vi "Excel报表.vi"() -> ()   [LabVIEW 2014]
uses:
  <vilib>/Utility/NIReport.llb/NI_report.lvclass
  <vilib>/Utility/NIReport.llb/Excel/NI_Excel.lvclass
panel:
  in  "template (empty)":path caption="模板（空）"
  in  "Relative Humidity":dbl[][](array[numeric])=[[0.54, 0.65, 0.56, 0.5, 0.45]]
  in  "Has Legend?":bool
  in  "Graph Type":i32(ring)=51 items=["xlColumnClustered"=51, "xlColumnStacked"=52, "xlColumnStacked100"=53, "xl3DColumnClustered"=54, "xl3DColumnStacked"=55, "xl3DColumnStacked100"=56, "xlBarClustered"=57, "xlBarStacked"=58, "xlBarStacked100"=59, "xl3DBarClustered"=60, "xl3DBarStacked"=61, "xl3DBarStacked100"=62, "xlLineStacked"=63, "xlLineStacked100"=64, "xlLineMarkers"=65, "xlLineMarkersStacked"=66, "xlLineMarkersStacked100"=67, "xlPieOfPie"=68, "xlPieExploded"=69, "xl3DPieExploded"=70, "xlBarOfPie"=71, "xlXYScatterSmooth"=72, "xlXYScatterSmoothNoMarkers"=73, "xlXYScatterLines"=74, "xlXYScatterLinesNoMarkers"=75, "xlAreaStacked"=76, "xlAreaStacked100"=77, "xl3DAreaStacked"=78, "xl3DAreaStacked100"=79, "xlDoughnutExploded"=80, "xlRadarMarkers"=81, "xlRadarFilled"=82, "xlSurface"=83, "xlSurfaceWireframe"=84, "xlSurfaceTopView"=85, "xlSurfaceTopViewWireframe"=86, "xlBubble"=15, "xlBubble3DEffect"=87, "xlStockHLC"=88, "xlStockOHLC"=89, "xlStockVHLC"=90, "xlStockVOHLC"=91, "xlCylinderColClustered"=92, "xlCylinderColStacked"=93, "xlCylinderColStacked100"=94, "xlCylinderBarClustered"=95, "xlCylinderBarStacked"=96, "xlCylinderBarStacked100"=97, "xlCylinderCol"=98, "xlConeColClustered"=99, "xlConeColStacked"=100, "xlConeColStacked100"=101, "xlConeBarClustered"=102, "xlConeBarStacked"=103, "xlConeBarStacked100"=104, "xlConeCol"=105, "xlPyramidColClustered"=106, "xlPyramidColStacked"=107, "xlPyramidColStacked100"=108, "xlPyramidBarClustered"=109, "xlPyramidBarStacked"=110, "xlPyramidBarStacked100"=111, "xlPyramidCol"=112, "xl3DColumn"=-4100, "xlLine"=4, "xl3DLine"=-4101, "xl3DPie"=-4102, "xlPie"=5, "xlXYScatter"=-4169, "xl3DArea"=-4098, "xlArea"=1, "xlDoughnut"=-4120, "xlRadar"=-4151]
  in  "Month":string[](array[string])=["Jan", "Feb", "Mar", "Apr", "May"]
  in  "Window State":enum16{"maximized", "minimized", "normal"}(ring)
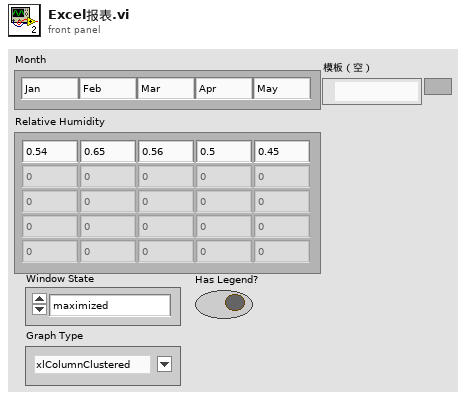
[diagram p1: front panel]
types:
  T1 = enum16{"maximized", "minimized", "normal", "no change"}
  T2 = cluster{"font style":string, "bold":bool, "italic":bool, "underline":bool, "size":sgl, "color":u32}
  T3 = cluster{"left":i32, "top":i32, "height":dbl, "width":dbl}
  T4 = enum16{"Standard Report", "HTML", "Word", "Excel"}
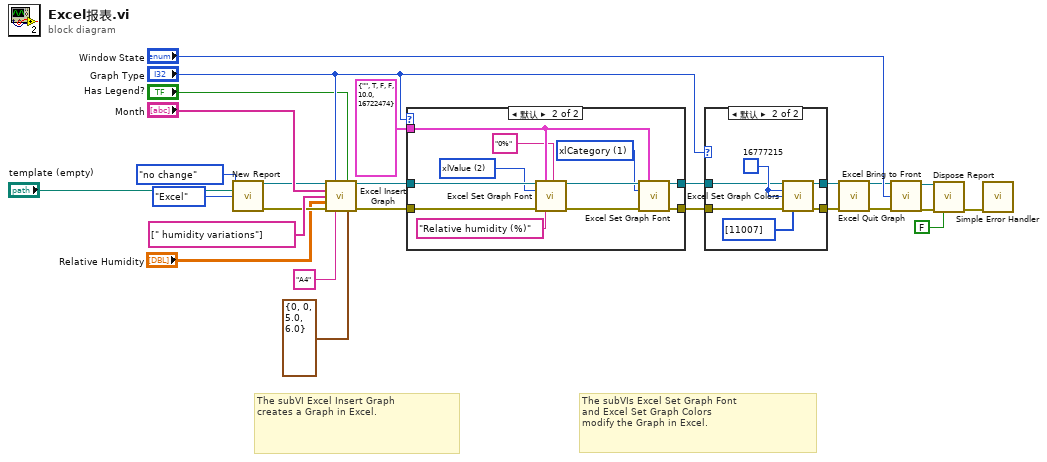
[diagram p0: block diagram]
diagram:
  # "The subVIs Excel Set Graph Font \nand Excel Set Graph Colors \nmodify the Graph in Excel."
  # "The subVI Excel Insert Graph \ncreates a Graph in Excel."
  n1 = call <vilib>:"New Report.vi"("window state (normal)"=T1."no change", "report type"=T4."Excel", "template (empty)"="template (empty)") -> ("report out"=w13:refnum<class "NI_report.lvclass">, "error out"=w12:errorcluster)  [unwired: 11 in]
  n2 = call <vilib>:"Excel Insert Graph.vi"("report in"=w13, "graph type (col clustered)"="Graph Type", "has legend? (F)"="Has Legend?", "column headers"="Month", "row headers"=string[] [" humidity variations"], "data"="Relative Humidity", "error in (no error)"=w12, "name (\"\")"="A4" ("name (\"\")"), "position/size"=T3 {"left"=0, "top"=0, "height"=5.0, "width"=6.0}) -> ("report out"=w5:refnum<class "NI_report.lvclass">, "error out"=w6:errorcluster)  [unwired: 5 in]
  n3 = case shown="默认" "Graph Type" {
    tunnel: w5 -> [w28 w39]
    tunnel: w6 -> [w27 w38]
    tunnel: [w28 w36] -> w8
    tunnel: [w27 w35] -> w7
    tunnel: T2 {"font style"="", "bold"=TRUE, "italic"=FALSE, "underline"=FALSE, "size"=10.0, "color"=16722474} ("axis font") -> [_ w30]
    frame -4151, -4120, -4102, 5, 68..71, 80..82 {
      # "These Graph Types are not supported"
    }
    frame Default {
      w33 = 2 items=["xlCategory"=1, "xlSeriesAxis"=3, "xlValue"=2] ("type")
      w32 = 1 items=["xlCategory"=1, "xlSeriesAxis"=3, "xlValue"=2] ("type")
      n4 = call <vilib>:"Excel Set Graph Font.vi"("report in"=w39, "axis font"=w30, "number format (general)"="0%" ("number format (\"\")"), "axis type (xlCategory)"=w33, "error in (no error)"=w38, "title (\"\")"="Relative humidity (%)" ("title (\"\")")) -> ("report out"=w37:refnum<class "NI_report.lvclass">, "error out"=w34:errorcluster)  [unwired: 8 in]
      n5 = call <vilib>:"Excel Set Graph Font.vi"("report in"=w37, "axis font"=w30, "axis type (xlCategory)"=w32, "error in (no error)"=w34) -> ("report out"=w36:refnum<class "NI_report.lvclass">, "error out"=w35:errorcluster)  [unwired: 10 in]
    }
  }
  n6 = case shown="默认" "Graph Type" {
    tunnel: w8 -> [w41 w45]
    tunnel: w7 -> [w40 w44]
    tunnel: [w41 w43] -> w9
    tunnel: [w40 w42] -> w10
    frame 15, 87 {
    }
    frame Default {
      w46 = u32 16777215 ("plot area color")
      n7 = call <vilib>:"Excel Set Graph Colors.vi"("report in"=w45, "graph area color (w)"=w46, "plot area color (w)"=w46, "error in (no error)"=w44, "plot colors"=u32[] [11007]) -> ("report out"=w43:refnum<class "NI_report.lvclass">, "error out"=w42:errorcluster)  [unwired: 9 in]
    }
  }
  n8 = call <vilib>:"Excel Quit Graph.vi"("report in"=w9, "error in (no error)"=w10) -> ("report out"=w17:refnum<class "NI_report.lvclass">, "error out"=w18:errorcluster)  [unwired: 12 in]
  n9 = call <vilib>:"Excel Bring to Front.vi"("report in"=w17, "window state (maximized)"="Window State", "error in (no error)"=w18) -> ("report out"=w14:refnum<class "NI_report.lvclass">, "error out"=w16:errorcluster)  [unwired: 11 in]
  n10 = call-dynamic "Dispose Report.vi"("report in"=w14, "error in (no error)"=w16, "close report? (T)"=FALSE ("Close Report? (T)")) -> ("error out"=w26:errorcluster)  [unwired: 12 in]
  n11 = call <vilib>:"Simple Error Handler.vi"("error in (no error)"=w26) -> ()  [unwired: 4 in, 5 out]
